vi "QueueNames.vi"(8 "error in (no error)":errorcluster) -> (0 "error out":errorcluster, 2 "Queue Names":string[](array[string]))   [LabVIEW 2017, in "MDPtr.lvlib" / "MDPtrMgr.lvclass"]
uses:
  MDPtrMgr.lvclass
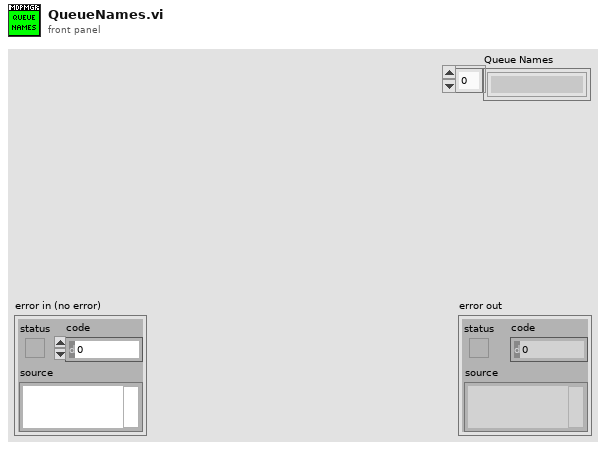
[diagram p1: front panel]
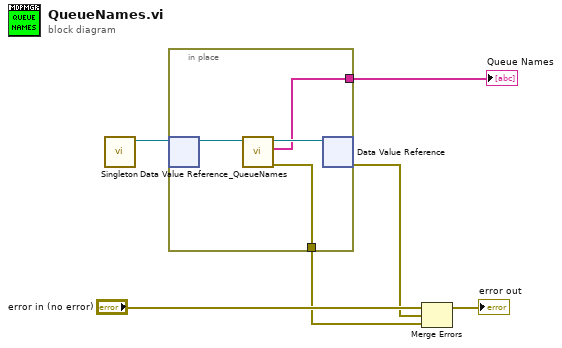
[diagram p0: block diagram]
diagram:
  n1 = call "Singleton.vi"() -> ("MDPtrMgrDVR"=w6:refnum<data-value>)  [unwired: 10 in, 1 out]
  n2 = in-place {
    in-place-border: [w8] -> w2
    in-place-border: [w7] -> w1
    n3 = in-place-dvr #1(w6) -> (w10:refnum<class "MDPtrMgr.lvclass">)  [unwired: 1 out]
    n4 = call "_QueueNames.vi"("MDPtrMgr in"=w10) -> ("error out"=w8:errorcluster, "Queue Names"=w7:string[], "MDPtrMgr out"=w9:refnum<class "MDPtrMgr.lvclass">)  [unwired: 8 in]
    n5 = in-place-dvr #1(w9) -> (w3:errorcluster)  [unwired: 1 out]
  }
  "Queue Names" <- w1
  n6 = Merge Errors("error in (no error)", w3, w2) -> (→"error out":errorcluster)
